vi "WhiteScreenTest_Startup.vi"() -> (0 "ErrorOut":errorcluster)   [LabVIEW 2018] (continued)
        n220 = Enqueue Element(queue=w531, element=cluster{"QElmnt":T47, "Data":variant} {"QElmnt"=enum."Spvsr_RfrshPnl", "Data"=variant} ("Cluster"), error in (no error)=w530) -> (error out=w529:errorcluster)  [unwired: 3 out]
        n221 = Variant To Data(error in=w529, type=w529, Variant=w532) -> (data=w533:errorcluster, error out=w525:errorcluster)
        n222 = Unbundle By Name(w533) -> ("code"=w526:i32)
        n223 = call "CheckForExistingErrorDialog.vi"("ErrorIn"=w525, "ErrorCodeIn"=w526) -> ("ErrorOut"=w523:errorcluster, "NoWndwFnd"=w522:bool, "ErrorCodeOut"=w524:i32)  [unwired: 7 in]
        n224 = call "PushToErrorHandler.vi"("ErrorIn"=w523, "ErrorLocation"="Error Handler") -> ("ErrorOut"=w538:errorcluster)  [unwired: 5 in]
        n225 = case shown="True" w522 {
          tunnel: w538 -> [w539 w547]
          tunnel: [w539 w546] -> w537
          tunnel: w536 -> [_ w545]
          tunnel: w535 -> [w540 w544]
          tunnel: [w540 w543] -> w534
          tunnel: w533 -> [_ w542]
          tunnel: w524 -> [_ w541]
          frame False {
          }
          frame True {
            n226 = case shown="-8998" w541 {
              tunnel: [w555 w564 w566 w573 w577 w584 w593] -> w546
              tunnel: w544 -> [w551 w560 w567 w572 w579 w589 w591]
              tunnel: [w550 w559 w568 w572 w580 w583 w591] -> w543
              tunnel: w547 -> [w556 w565 w566 w571 w577 w585 w594]
              tunnel: w542 -> [w554 w563 _ w574 _ w586 w595]
              tunnel: w545 -> [_ _ _ _ _ _ _]
              frame Default {
                # "-1 dictates that the message box does NOT time out"
                # "Default Error Case handles all error codes undefined by this structure."
                n227 = Bundle By Name(cluster=w551, "Stat.SysState"=SystemStateEnum."System Fault") -> (w550:T32)
                n228 = Unbundle By Name(w550) -> ("SMS"=w549:T36)
                n229 = call "LaunchSystemMessageDialogBox.vi"("ErrorToProcess"=w554, "SMS"=w549, "ErrorIn"=w556, "CorrAct"="Undocumented System Error, please record this information and contact the vendor.", "Timeout(ms)"=-1 ("Timeout (-1)")) -> ("ErrorOut"=w555:errorcluster)  [unwired: 6 in]
              }
              frame -8998 {
                # "-1 dictates that the message box does NOT time out"
                # "Default Error Case handles all error codes undefined by this structure."
                n230 = Bundle By Name(cluster=w560, "Stat.SysState"=SystemStateEnum."System Fault") -> (w559:T32)
                n231 = Unbundle By Name(w559) -> ("SMS"=w558:T36)
                n232 = call "LaunchSystemMessageDialogBox.vi"("ErrorToProcess"=w563, "SMS"=w558, "ErrorIn"=w565, "CorrAct"="The FPGAs are configured for an external 10 MHz reference clock. It doesn't look like that clock is working right.", "Timeout(ms)"=-1 ("Timeout (-1)")) -> ("ErrorOut"=w564:errorcluster)  [unwired: 6 in]
              }
              frame 5000 {
                # "Example User Defined Error Code.  Disable the Hardware and no Dialog Box"
                n233 = Bundle By Name(cluster=w567, "Stat.SysState"=SystemStateEnum."System Fault") -> (w568:T32)
              }
              frame 5998 {
                n234 = Unbundle By Name(w572) -> ("SMS"=w575:T36)
                n235 = call "LaunchSystemMessageDialogBox.vi"("ErrorToProcess"=w574, "SMS"=w575, "ErrorIn"=w571, "CorrAct"="Error Log Failure\n\n- There was an error writing to the Error Log File, please verify that the current user has read/write permissions to the <Users>\\My Documents & the <Users>\\Desktop folders" ("CorrAction"), "Timeout(ms)"=-1) -> ("ErrorOut"=w573:errorcluster)  [unwired: 6 in]
              }
              frame 5999 {
                n236 = Bundle By Name(cluster=w579, "Stat.SysState"=SystemStateEnum."System Error") -> (w580:T32)
              }
              frame 5100..5149 {
                # "Disable Hardware?"
                # "These error codes are reserved for Config File Reads"
                n237 = Bundle By Name(cluster=w589, "Stat.SysState"=SystemStateEnum."System Fault") -> (w583:T32)
                n238 = Unbundle By Name(w583) -> ("SMS"=w582:T36)
                n239 = call "LaunchSystemMessageDialogBox.vi"("ErrorToProcess"=w586, "SMS"=w582, "ErrorIn"=w585, "CorrAct"="Configuration File Read Error\n\n- One or more Configuration File Fields were not found or improperly loaded.\n- All System Hardware has been disabled\n- Launch the Configuration Panels and verify that all values have been correctly entered\n- Reinitialize the Hardware" ("CorrAction"), "Timeout(ms)"=-1 ("Timeout")) -> ("ErrorOut"=w584:errorcluster)  [unwired: 6 in]
              }
              frame 5150..5199 {
                # "No need to disable hardware here"
                # "These error codes are reserved for Config File Writes"
                n240 = Unbundle By Name(w591) -> ("SMS"=w592:T36)
                n241 = call "LaunchSystemMessageDialogBox.vi"("ErrorToProcess"=w595, "SMS"=w592, "ErrorIn"=w594, "CorrAct"="Configuration File Write Error\n\n- One or more Configuration File Fields were not found or specified incorrectly.\n- Launch the Configuration Panels and verify that all values have been correctly entered" ("CorrAction"), "Timeout(ms)"=-1 ("Timeout")) -> ("ErrorOut"=w593:errorcluster)  [unwired: 6 in]
              }
            }
          }
        }
      }
      frame "Spvsr_Config" {
        # "Opens the Configuration Panel"
        n242 = Current VI's Path() -> (path=w602:path)
        n243 = call "SetVIWindowTransparency.vi"("VIPath"=w602, "ErrorIn"=w603) -> ("ErrorOut"=w601:errorcluster)  [unwired: 9 in]
        n244 = call "ConfigPanel.vi"("ErrorIn"=w601, "ClusterIn"=w604) -> ("ErrorOut"=w597:errorcluster, "ClusterOut"=w598:T32)  [unwired: 8 out]
        n245 = Current VI's Path() -> (path=w599:path)
        n246 = call "RestoreVIWindowTransparency.vi"("VIPath"=w599, "ErrorIn"=w597) -> ("ErrorOut"=w600:errorcluster)  [unwired: 9 in]
      }
      frame "Spvsr_FPConfig" {
        w647 = ScaleMeasure."50" ("ScaleMeasure")
        w644 = ext 1.0 ("Scale_In_RT")
        w645 = fxp<+/-,30,30> 536870911.0 ("Scale_NoiseFloor")
        # "Don't start other loops if paths are bad."
        n247 = disable-structure shown="Enabled" {
          disable-tunnel: w609 -> [w668 _]
          disable-tunnel: [w667 T41 {"#NoiseSums"=1, "Max_df"=1, "AvgAvg"=FALSE, "#Avg"=1, "AutoCenter"=FALSE, "Inclin"={"Vmin"=0.0, "Vmax"=0.0, "Angle_min"=0.0, "Angle_max"=0.0, "Offset"=0.0, "Pos_Neg"=FALSE}, "1"={"Cal_"={"Fine"=0.000213623046875, "Coarse_"=4194303.0}, "Beac"={"Fine"=4194303.0, "Coarse_"=1.0}, "Scale"={"Step4"=10000.0, "Step5"=4194303.0, "Step6"=1.0, "Step7"=10000.0}, "Offset"=0.0, "Scale_Noise"=4194303.0, "Scale_Step1"=65535.0, "Scale_In_RT"=1.0, "ScaleMeas"=0.999969482421875, "FreqsToRemove"=[0, 1633], "Width"=[0, 1633], "ScaleMeasEnum"=enum."50", "FilterEnab"=enum."Step 1"}, "2"={"Cal_"={"Fine"=0.000213623046875, "Coarse_"=4194303.0}, "Beac"={"Fine"=0.000213623046875, "Coarse_"=4194303.0}, "Scale"={"Step4"=0.0, "Step5"=4194303.0, "Step6"=1.0, "Step7"=10000.0}, "Offset"=0.0, "Scale_Noise"=4194303.0, "Scale_Step1"=65535.0, "Scale_In_RT"=1.0, "ScaleMeas"=0.999969482421875, "FreqsToRemove"=[0, 1633], "Width"=[0, 1633], "ScaleMeasEnum"=enum."50", "FilterEnab"=enum."Step 1"}, "3"={"Cal_"={"Fine"=0.000213623046875, "Coarse_"=4194303.0}, "Beac"={"Fine"=0.000213623046875, "Coarse_"=4194303.0}, "Scale"={"Step4"=0.0, "Step5"=4194303.0, "Step6"=1.0, "Step7"=10000.0}, "Offset"=0.0, "Scale_Noise"=4194303.0, "Scale_Step1"=65535.0, "Scale_In_RT"=1.0, "ScaleMeas"=0.999969482421875, "FreqsToRemove"=[0, 1633], "Width"=[0, 1633], "ScaleMeasEnum"=enum."50", "FilterEnab"=enum."Step 1"}, "4"={"Cal_"={"Fine"=0.000213623046875, "Coarse_"=4194303.0}, "Beac"={"Fine"=0.000213623046875, "Coarse_"=4194303.0}, "Scale"={"Step4"=0.0, "Step5"=4194303.0, "Step6"=1.0, "Step7"=10000.0}, "Offset"=0.0, "Scale_Noise"=4194303.0, "Scale_Step1"=1.0, "Scale_In_RT"=10000.0, "ScaleMeas"=0.999969482421875, "FreqsToRemove"=[0, 1633], "Width"=[0, 1633], "ScaleMeasEnum"=enum."50", "FilterEnab"=enum."Step 1"}, "Target to Probe"=enum."4", "SNR_Thresh"=1.0, "Paths"={"CfgFile"=path "", "LogFolder"=path "", "LogFile"=path "", "NAS path"=path "", "ThreshFile"=path "", "RedunFolder"=path ""}, "Connex_Location"="", "SimulateFPGA"=FALSE} ("FP_User")] -> w608
          frame Enabled {
            # "12/14/2020"
            n248 = Unbundle By Name(w668) -> ("Config.FP_User"=w667:T41)
          }
          frame Disabled {
          }
        }
        n249 = Unbundle By Name("Scale") -> ("Measure"=w631:fxp<+/-,16,1>, "Step1"=w632:fxp<+/-,17,17>, "Scale"=w633:T5)
        n250 = call "RootExists.vi"("path"="NAS path") -> ("file or folder exists?"=w611:bool)  [unwired: 10 in]
        n251 = Negate(x="Shift Cal") -> (-x=w626:T11)
        n252 = Negate(x="Shift Beac") -> (-x=w625:T11)
        n253 = Not(x=w611) -> (.not. x?=→"Logging to NAS":bool)
        n254 = Bundle By Name(cluster=w608, "1.ScaleMeas"=w631, "1.Scale_Step1"=w632, "1.Scale"=w633, "1.ScaleMeasEnum"=w647, "AvgAvg"="AvgAvg", "1.FreqsToRemove"="FreqsToRemove", "1.Width"="Width [bins]", "1.Cal_"=w626, "1.Beac"=w625, "1.FilterEnab"="FilterEnable", "1.Scale_Noise"=w645, "1.Scale_In_RT"=w644, "#NoiseSums"=u32 86400 ("#NoiseSums to log"), "AutoCenter"="AutoCenter", "Target to Probe"="Target to Probe", "#Avg"=u16 150 ("#Avg in FPGA"), "SNR_Thresh"="SNR_Thresh", "Inclin"="Inclin", "Paths.RedunFolder"="base path", "Paths.LogFolder"="base path", "Paths.NAS path"="NAS path", "Paths.ThreshFile"="ThreshFile", "Connex_Location"="Location", "Max_df"="MaxTrackRate", "SimulateFPGA"="SimulateFPGA") -> (w656:T41)
        n255 = Build Array("base path", "ThreshFile") -> (w629:path[])
        n256 = Select(t=enum32{"Auto", "Manual"}."Auto" ("FreqShiftTab"), s="AutoCenter", f=enum32{"Auto", "Manual"}."Manual" ("FreqShiftTab")) -> (s? t:f=→"FreqShiftTab_72Co" →"FreqShiftTab_84Co":enum32{"Auto", "Manual"})
        n257 = for {
          tunnel: w629 -> [w679] mode=indexing
          tunnel: [w677] -> w628 mode=indexing
          n258 = call "RootDoesntExist.vi"("base path in"=w679) -> ("String"=w678:string)  [unwired: 10 in]
          n259 = call "RootExists.vi"("path"=w679) -> ("file or folder exists?"=w677:bool)  [unwired: 10 in]
          n260 = case shown="False" w677 {
            tunnel: w678 -> [w680 _]
            frame False {
              n261 = One Button Dialog(message=w680) -> ()  [unwired: 1 in, 1 out]
            }
            frame True {
            }
          }
        }
        n262 = Unbundle By Name(w656) -> ("2"=w655:T42)
        n263 = Bundle By Name(cluster=w655, "ScaleMeas"=w631, "Scale_Step1"=w632, "Scale"=w633, "ScaleMeasEnum"=w647, "FreqsToRemove"="FreqsToRemove", "Width"="Width [bins]", "FilterEnab"="FilterEnable", "Scale_Noise"=w645, "Scale_In_RT"=w644, "Cal_"=w626, "Beac"=w625) -> (w657:T42)
        n264 = Bundle By Name(cluster=w656, "2"=w657) -> (w650:T41)
        n265 = Negate(x="Shift Cal 3") -> (-x=w624:T11)
        n266 = Negate(x="Shift Beac 3") -> (-x=w623:T11)
        n267 = Unbundle By Name(w650) -> ("3"=w654:T42)
        n268 = Bundle By Name(cluster=w654, "ScaleMeas"=w631, "Scale_Step1"=w632, "Scale"=w633, "ScaleMeasEnum"=w647, "FreqsToRemove"="FreqsToRemove 2", "Width"="Width 2 [bins]", "FilterEnab"="FilterEnable", "Scale_Noise"=w645, "Scale_In_RT"=w644, "Cal_"=w624, "Beac"=w623) -> (w653:T42)
        n269 = And Array Elements(Boolean array=w628) -> (logical AND=w627:bool)
        n270 = Bundle By Name(cluster=w650, "3"=w653) -> (w649:T41)
        n271 = Unbundle By Name(w649) -> ("4"=w651:T42)
        n272 = Bundle By Name(cluster=w651, "ScaleMeas"=w631, "Scale_Step1"=w632, "Scale"=w633, "ScaleMeasEnum"=w647, "FreqsToRemove"="FreqsToRemove 2", "Width"="Width 2 [bins]", "FilterEnab"="FilterEnable", "Scale_Noise"=w645, "Scale_In_RT"=w644, "Cal_"=w624, "Beac"=w623) -> (w652:T42)
        n273 = Bundle By Name(cluster=w649, "4"=w652) -> (w648:T41)
        n274 = Bundle By Name(cluster=w609, "Config.FP_User"=w648) -> (w619:T32)
        n275 = Bundle By Name(cluster=w619, "Config.FP_User.Max_df"=u32 1) -> (w618:T32)
        n276 = case shown="True" w627 {
          tunnel: w666 -> [w670 w676]
          tunnel: w619 -> [_ w671]
          tunnel: w664 -> [_ w675]
          tunnel: [w670 w674] -> w660
          tunnel: w659 -> [_ w673]
          tunnel: w635 -> [_ w672]
          frame False {
          }
          frame True {
            n277 = call "Send_Front_Panel_Config_to_Loops.vi"("ClusterIn"=w671, "Log_Q"=w672, "error in (no error)"=w676, "Noise_Q"=w673, "Tones_Q"=w675) -> ("error out"=w674:errorcluster)  [unwired: 6 in]
          }
        }
        n278 = call "WriteConfigFile.vi"("ErrorIn"=w660, "ClusterIn"=w618) -> ("ErrorOut"=w665:errorcluster)  [unwired: 1 in, 8 out]
        "Auto Center" <- "AutoCenter"
      }
      frame "Spvsr_AlarmCfg" {
        # "We send alarm configurations to AI and TC. The voltage and\ntemp indicators are color-coded red & yellow if there are \nalarms or wanings. These are calculated in the AI loops."
        # "We need to send the alarm configuration to the log loop because that is\nwhere we will check the alarm statuses. It's the only place where we can find\nthe data from AI, TC, TE, ADAM, and spectra."
        n279 = Unbundle By Name(w693) -> ("Config.FP_User.Paths.ThreshFile"=w692:path)
        n280 = Bundle By Name(cluster=w693, "Alarm"="AlarmSettings") -> (w696:T32)
        n281 = Flatten To XML(anything="AlarmSettings") -> (xml string=w695:string)
        n282 = call-poly <vilib>:"Write to XML File.vi"("error in (no error)"=w694, "XML Input"=w695, "XML File Path"=w692) -> ("error out"=w691:errorcluster)  [unwired: 6 in, 2 out]
        n283 = To Variant(anything="AlarmSettings") -> (Variant=w682:variant)
        n284 = To Variant(anything="AlarmSettings") -> (Variant=w686:variant)
        n285 = Bundle By Name(cluster=cluster{"Enum":T30, "Data":variant} {"Enum"=enum."Log_CfgAlarm", "Data"=variant} ("element"), "Data"=w686) -> (w687:cluster{"Enum":T30, "Data":variant})
        n286 = Bundle By Name(cluster=cluster{"Enum":T53, "Var":variant} {"Enum"=enum."AI_Alarm", "Var"=variant}, "Var"=w682) -> (w683:cluster{"Enum":T53, "Var":variant})
        n287 = Enqueue Element(queue=w689, element=w687, error in (no error)=w691) -> (error out=w690:errorcluster)  [unwired: 1 in, 2 out]
        n288 = for {
          tunnel: string[] ["AI", "TC"] ("name (unnamed)") -> [w704] mode=indexing
          tunnel: w683 -> [w697]
          n289 = Obtain Queue(max queue size (-1, unlimited)=100, name (unnamed)=w704, element data type=w697) -> (queue out=w702:refnum<queue>, error out=w703:errorcluster)  [unwired: 2 in, 1 out]
          n290 = Enqueue Element(queue=w702, element=w697, error in (no error)=w703) -> (queue out=w700:refnum<queue>, error out=w701:errorcluster)  [unwired: 1 in, 1 out]
          n291 = Release Queue(queue=w700, error in (no error)=w701) -> (error out=w699:errorcluster)  [unwired: 1 in, 2 out]
          n292 = call "PushToErrorHandler.vi"("ErrorIn"=w699, "ErrorLocation"="SendAlarmToAI_orTC") -> ()  [unwired: 5 in, 1 out]
        }
      }
      frame "Spvsr_DigitzOffs" {
        w714 = fxp<+/-,16,16> 0.0 ("fixed-point type")
        n293 = local read "84 GHz"() -> (w722:T3)
        n294 = local read "72 GHz"() -> (w723:T3)
        n295 = Unbundle By Name(w723) -> ("MeasMean0"=w719:dbl, "MeasMean1"=w717:dbl)
        n296 = Unbundle By Name(w722) -> ("MeasMean0"=w716:dbl, "MeasMean1"=w715:dbl)
        n297 = Negate(x=w719) -> (-x=w709:dbl)
        n298 = Negate(x=w717) -> (-x=w708:dbl)
        n299 = Negate(x=w716) -> (-x=w707:dbl)
        n300 = Negate(x=w715) -> (-x=w706:dbl)
        n301 = To Fixed-Point(fixed-point type=w714, number=w709) -> (fixed-point=w718:fxp<+/-,16,16>)
        "Digitizer Offset 72 Co" <- w718
        n302 = To Fixed-Point(fixed-point type=w714, number=w708) -> (fixed-point=w712:fxp<+/-,16,16>)
        "Digitizer Offset 72 X" <- w712
        n303 = To Fixed-Point(fixed-point type=w714, number=w707) -> (fixed-point=w711:fxp<+/-,16,16>)
        "Digitizer Offset 84 Co" <- w711
        n304 = To Fixed-Point(fixed-point type=w714, number=w706) -> (fixed-point=w710:fxp<+/-,16,16>)
        "Digitizer Offset 84 x" <- w710
        n305 = Bundle By Name(cluster=w720, "Config.FP_User.1.Offset"=w718, "Config.FP_User.2.Offset"=w712, "Config.FP_User.3.Offset"=w711, "Config.FP_User.4.Offset"=w710) -> (w721:T32)
      }
      frame "FP_AO_ctrl" {
        w746 = 5.0
        w747 = 0.0
        w741 = cluster{"Enum":T55, "Data":variant} {"Enum"=enum."AO_Write", "Data"=variant}
        # "As defined in Wiring_Pinout Diagrams_DRAFT_20171207.xlsx\nfrom Nick Tarasenko.\nLuke 12-12-2017"
        # "Cal tones: 5 is on, 0 is off"
        # "Noise: 0 is on, 5 is off"
        n306 = Select(t=w747, s="noise_ctrl", f=w746) -> (s? t:f=w745:dbl)
        n307 = Select(t=w746, s="72GHz_ctrl", f=w747) -> (s? t:f=w744:dbl)
        n308 = Select(t=w746, s="84GHz_ctrl", f=w747) -> (s? t:f=w743:dbl)
        n309 = Obtain Queue(max queue size (-1, unlimited)=100, name (unnamed)="AO", element data type=w741, error in (no error)=w748) -> (queue out=w751:refnum<queue>, error out=w737:errorcluster)  [unwired: 1 in, 1 out]
        n310 = Build Array("noise_ctrl", "72GHz_ctrl", "84GHz_ctrl") -> (w726:bool[])
        n311 = Build Array(w745, w744, w743) -> (w742:dbl[])
        n312 = To Variant(anything=w742) -> (Variant=w730:variant)
        n313 = Bundle By Name(cluster=w741, "Data"=w730) -> (w740:cluster{"Enum":T55, "Data":variant})
        n314 = Enqueue Element(queue=w751, element=w740, error in (no error)=w737) -> (queue out=w736:refnum<queue>, error out=w738:errorcluster)  [unwired: 1 in, 1 out]
        n315 = To Variant(anything=w726) -> (Variant=w725:variant)
        n316 = Release Queue(queue=w736, error in (no error)=w738) -> (error out=w735:errorcluster)  [unwired: 1 in, 2 out]
        n317 = Bundle By Name(cluster=cluster{"Enum":T30, "Data":variant} {"Enum"=enum."Log_DO", "Data"=variant} ("element"), "Data"=w725) -> (w731:cluster{"Enum":T30, "Data":variant})
        n318 = Enqueue Element(queue=w733, element=w731, timeout in ms (-1)=10, error in (no error)=w735) -> (error out=w734:errorcluster)  [unwired: 2 out]
      }
      frame "Spvsr_ScaleGraphs" {
        w786 = 1000000.0 ("y")
        w783 = 10.0 ("y")
        # "This was a local variable tied to Frequency Shift Enable, before the control was changed to a constant. Luke 6-1-2018"
        n319 = local read "BeaconShift 3"() -> (w765:dbl)
        n320 = local read "BeaconShift 2"() -> (w799:dbl)
        n321 = local read "BeaconShift 4"() -> (w763:dbl)
        n322 = local read "BeaconShift"() -> (w795:dbl)
        n323 = local read "Peak Location Beacon"() -> (w781:dbl)
        n324 = local read "Peak Location Cal"() -> (w782:dbl)
        n325 = local read "Peak Location Beacon 2"() -> (w801:dbl)
        n326 = local read "Peak Location Cal 2"() -> (w802:dbl)
        n327 = local read "Peak Location Beacon 3"() -> (w761:dbl)
        n328 = local read "Peak Location Cal 3"() -> (w760:dbl)
        n329 = local read "Peak Location Beacon 4"() -> (w759:dbl)
        n330 = local read "Peak Location Cal 4"() -> (w758:dbl)
        n331 = local read "CalShift 3"() -> (w764:dbl)
        n332 = local read "CalShift 2"() -> (w800:dbl)
        n333 = local read "CalShift"() -> (w796:dbl)
        n334 = local read "CalShift 4"() -> (w762:dbl)
        n335 = control-ref of="NoiseFloor"() -> (w756:refnum<vi>)
        n336 = control-ref of="NoiseFloor 2"() -> (w754:refnum<vi>)
        n337 = control-ref of="NoiseFloor 3"() -> (w753:refnum<vi>)
        n338 = control-ref of="NoiseFloor 4"() -> (w752:refnum<vi>)
        n339 = local read "df (Hz)"() -> (w777:dbl)
        n340 = Build Array(w795, w796, w799, w800, w765, w764, w763, w762) -> (w790:dbl[])
        n341 = Build Array(w756, w754, w753, w752) -> (w755:refnum<vi>[])
        n342 = for {
          tunnel: [w833] -> w772
          tunnel: w790 -> [w835] mode=indexing
          tunnel: TRUE -> [w829]
          tunnel: [w828] -> w771 mode=indexing
          n343 = local read "df (Hz)"() -> (w836:dbl)
          n344 = Divide(x=w836, y=1000000.0) -> (x/y=w833:dbl)
          n345 = Divide(x=w835, y=1000000.0) -> (x/y=w831:dbl)
          n346 = Select(t=w831, s=w829, f=0.0) -> (s? t:f=w828:dbl)
        }
        n347 = Build Array(w781, w782, w801, w802, w761, w760, w759, w758) -> (w791:dbl[])
        n348 = for {
          tunnel: w777 -> [w805]
          tunnel: u8 0 ("Noise Floor") -> [w804]
          tunnel: w755 -> [w803] mode=indexing
          n349 = property class="WFGraph (strict)"(reference=w803, "YScale.Mapping Mode"=w804, "XScale.Multiplier"=w805) -> ()  [unwired: 1 in, 2 out]
        }
        n350 = case shown="True" "AutoScale Y Noise" {
          tunnel: w755 -> [_ w806]
          frame False {
          }
          frame True {
            n351 = for {
              tunnel: w806 -> [w808] mode=indexing
              n352 = property class="WFGraph (strict)"(reference=w808, "YScale.ScaleFit"=u8 1 ("Y Scale.Scale Fit")) -> ()  [unwired: 1 in, 2 out]
            }
          }
        }
        n353 = Add(x=w791, y=w783) -> (x+y=w784:dbl[])
        n354 = Subtract(x=w791, y=w783) -> (x-y=w785:dbl[])
        n355 = Divide(x=w784, y=w786) -> (x/y=w788:dbl[])
        n356 = Divide(x=w785, y=w786) -> (x/y=w789:dbl[])
        n357 = control-ref of="All Spectrums"() -> (w773:refnum<vi>)
        n358 = Index Array(array=w771) -> (element=w770:dbl)  [unwired: 1 in]
        n359 = control-ref of="Beacon 2"() -> (w797:refnum<vi>)
        n360 = control-ref of="Cal 2"() -> (w798:refnum<vi>)
        n361 = control-ref of="Beacon 3"() -> (w769:refnum<vi>)
        n362 = control-ref of="Beacon"() -> (w780:refnum<vi>)
        n363 = control-ref of="Cal"() -> (w778:refnum<vi>)
        n364 = control-ref of="Cal 3"() -> (w768:refnum<vi>)
        n365 = control-ref of="Cal 4"() -> (w766:refnum<vi>)
        n366 = control-ref of="Beacon 4"() -> (w767:refnum<vi>)
        n367 = property class="WFGraph (strict)"(reference=w773, "XScale.Multiplier"=w772, "XScale.Offset"=w770) -> ()  [unwired: 1 in, 2 out]
        n368 = Build Array(w780, w778, w797, w798, w769, w768, w767, w766) -> (w792:refnum<vi>[])
        n369 = for {
          tunnel: w792 -> [w840] mode=indexing
          tunnel: u8 0 ("Tones") -> [w839]
          tunnel: w772 -> [w838]
          tunnel: w771 -> [w837] mode=indexing
          n370 = property class="WFGraph"(reference=w840, "YScale.Mapping Mode"=w839, "XScale.Multiplier"=w838, "XScale.Offset"=w837) -> ()  [unwired: 1 in, 2 out]
        }
        n371 = for {
          tunnel: w792 -> [w816] mode=indexing
          tunnel: "Zoom On Peak" -> [w815]
          tunnel: w788 -> [w814] mode=indexing
          tunnel: w789 -> [w813] mode=indexing
          tunnel: [w812] -> _
          n372 = case shown="True" w815 {
            tunnel: w816 -> [w821 w823]
            tunnel: w814 -> [w819 _]
            tunnel: w813 -> [w818 _]
            tunnel: [w817 w822] -> w812
            frame True {
              n373 = property class="WFGraph"(reference=w821, "XScale.ScaleFit"=u8 0 ("X Scale.Scale Fit"), "XScale.Maximum"=w819, "XScale.Minimum"=w818) -> (error out=w817:errorcluster)  [unwired: 1 in, 1 out]
            }
            frame False {
              n374 = disable-structure shown="Disabled" {
                disable-tunnel: w823 -> [w826 _]
                disable-tunnel: [w824 errorcluster {"status"=FALSE, "code"=0, "source"=""} ("error out")] -> w822
                frame Enabled {
                  n375 = property class="WFGraph"(reference=w826, "XScale.ScaleFit"=u8 2 ("X Scale.Scale Fit")) -> (error out=w824:errorcluster)  [unwired: 1 in, 1 out]
                }
                frame Disabled {
                }
              }
            }
          }
        }
        n376 = case shown="True" "AutoScale Y Tones" {
          tunnel: w792 -> [_ w809]
          frame False {
          }
          frame True {
            n377 = for {
              tunnel: w809 -> [w810] mode=indexing
              n378 = property class="WFGraph"(reference=w810, "YScale.ScaleFit"=u8 1 ("Y Scale.Scale Fit")) -> ()  [unwired: 1 in, 2 out]
            }
          }
        }
      }
      frame "Spvsr_TrackRate" {
        n379 = Bundle By Name(cluster=w842, "Stat.TrackRate"=FALSE) -> (w843:T32)
      }
      frame "Spvsr_AutoCenter" {
        w845 = FALSE  # Stat.AutoCentr
        n380 = Bundle By Name(cluster=w846, "Stat.AutoCentr"=w845) -> (w847:T32)
      }
      frame "Spvsr_RestartWarn" {
        n381 = One Button Dialog(message="When changing file paths, the change will not be implemented until the program is restarted.\n\nWhen changing the \"Connex Location\", the change will not be written to the data log header until a new file is made (either at midnight, or upon restarting.)") -> ()  [unwired: 1 in, 1 out]
      }
      frame "Spvsr_ChkTime" {
        # "Reset peak tracker to default 10 minutes after user changes it."
        n382 = Unbundle By Name(w866) -> ("Stat.AutoCentr"=w858:bool, "Stat.TrackRate"=w868:bool)
        n383 = call "Elapsed Time4"("Time Target (s)"=600.0, "Reset"=w868, "error in (no error)"=w869) -> ("Elapsed Time (s)"=w864:dbl, "Time has Elapsed"=w867:bool, "error out"=w865:errorcluster)  [unwired: 9 in, 5 out]
        n384 = case shown="True" w867 {
          tunnel: w866 -> [w887 w895]
          tunnel: [w887 w894] -> w855
          tunnel: w865 -> [w888 w892]
          tunnel: [w888 w889] -> w857
          tunnel: w864 -> [_ _]
          frame False {
          }
          frame True {
            n385 = control-ref of="MaxTrackRate"() -> (w891:refnum<vi>)
            n386 = property class="DigNum (strict)"(reference=w891, error in=w892, "Val(Sgnl)"=u32 1 ("Value (Signaling)")) -> (error out=w889:errorcluster)  [unwired: 1 out]
            n387 = Bundle By Name(cluster=w895, "Stat.TrackRate"=TRUE) -> (w894:T32)
          }
        }
        n388 = call "Elapsed Time5"("Time Target (s)"=600.0, "Reset"=w858, "error in (no error)"=w857) -> ("Elapsed Time (s)"=w861:dbl, "Time has Elapsed"=w859:bool, "error out"=w860:errorcluster)  [unwired: 9 in, 5 out]
        n389 = case shown="True" w859 {
          tunnel: w855 -> [w878 w886]
          tunnel: [w878 w885] -> w854
          tunnel: w860 -> [w879 w883]
          tunnel: [w879 w881] -> w856
          tunnel: w861 -> [_ _]
          frame False {
          }
          frame True {
            n390 = control-ref of="AutoCenter"() -> (w882:refnum<vi>)
            n391 = property class="Bool (strict)"(reference=w882, error in=w883, "Val(Sgnl)"=TRUE ("Value (Signaling)")) -> (error out=w881:errorcluster)  [unwired: 1 out]
            n392 = Bundle By Name(cluster=w886, "Stat.AutoCentr"=TRUE ("Stat.TrackRate")) -> (w885:T32)
          }
        }
        n393 = call "Elapsed Time3"("Time Target (s)"=2.0, "error in (no error)"=w856) -> ("Time has Elapsed"=w875:bool, "error out"=w852:errorcluster)  [unwired: 10 in, 6 out]
        n394 = Select(t=cluster{"QElmnt":T47, "Data":variant}[] [{"QElmnt"=enum."Spvsr_ScaleGraphs", "Data"=variant}, {"QElmnt"=enum."Spvsr_ChkTime", "Data"=variant}], s=w875, f=cluster{"QElmnt":T47, "Data":variant}[] [{"QElmnt"=enum."Spvsr_ChkTime", "Data"=variant}]) -> (s? t:f=w877:cluster{"QElmnt":T47, "Data":variant}[])
        n395 = for {
          tunnel: w877 -> [w898] mode=indexing
          tunnel: w876 -> [w897]
          shift-right: [w896] -> w872
          shift-left: _ -> [_]
          n396 = Enqueue Element(queue=w897, element=w898) -> (error out=w896:errorcluster)  [unwired: 2 in, 2 out]
        }
        n397 = Wait Until Next ms Multiple(millisecond multiple=u32 100 ("milliseconds to wait")) -> ()  [unwired: 1 out]
        n398 = Merge Errors(w872, w852) -> (w853:errorcluster)
      }
      frame "Spvsr_About" {
        # "Pops up the About dialog box where you can enter version, customer, contact and any other information regarding the application."
        n399 = call "About.vi"("error in"=w902, "Timeout (ms)"=5000) -> ("error out"=w901:errorcluster)  [unwired: 9 out]
      }
      frame "Spvsr_Exit" {
        # "With the Exit Button, we exit this loop and push the HW Loops to close."
        n400 = call "Exit_All_Loops.vi"("error in (no error)"=w904, "10Hz_Q"=w903, "Noise_Q"=w906, "Tones_Q"=w907) -> ("error out"=w905:errorcluster)  [unwired: 7 in]
      }
    }
    "SPVSR_Count" <- w292
  }
  n401 = while {
    tunnel: w70 -> [w911]
    tunnel: w98 -> [w922]
    tunnel: [w916] -> w133
    shift-right: [w915] -> _
    shift-left: T24 {"Alarms"={"Green"=FALSE, "Rx_Yell"=FALSE, "Cx_Yell"=FALSE, "Red"=FALSE, "Source"=""}, "Spectrum 1"=[], "Spectrum 2"=[], "Spectrum 3"=[], "Spectrum 4"=[], "HistoryWeighting"=0.0, "NoiseFloorSums"={"1"=0.0, "2"=0.0, "3"=0.0, "4"=0.0}, "PwrHist"={"72Co"={"Cal"=0.0, "Cal Smooth"=0.0, "Beac"=0.0, "Beac Smooth"=0.0, "NoiseFloorSum"=0.0, "NoiseFloorSum Smooth"=0.0}, "72X"={"Cal"=0.0, "Cal Smooth"=0.0, "Beac"=0.0, "Beac Smooth"=0.0, "NoiseFloorSum"=0.0, "NoiseFloorSum Smooth"=0.0}, "84Co"={"Cal"=0.0, "Cal Smooth"=0.0, "Beac"=0.0, "Beac Smooth"=0.0, "NoiseFloorSum"=0.0, "NoiseFloorSum Smooth"=0.0}, "84X"={"Cal"=0.0, "Cal Smooth"=0.0, "Beac"=0.0, "Beac Smooth"=0.0, "NoiseFloorSum"=0.0, "NoiseFloorSum Smooth"=0.0}}} -> [w914]
    tunnel: w92 -> [w913]
    i -> [w912]
    stop <- w917 stop-if-true
    # "Front panel updates"
    n402 = call "PushToErrorHandler.vi"("ErrorIn"=w922, "ErrorLocation"="FP") -> ("ErrorOut"=w924:errorcluster)  [unwired: 5 in]
    n403 = Get Queue Status(queue=w911) -> (# elements in queue=→"# in FP queue":i32)  [unwired: 2 in, 7 out]
    n404 = Dequeue Element(queue=w911, error in (no error)=w924) -> (queue out=w918:refnum<queue>, element=w923:cluster{"Enum":T28, "Data":variant}, error out=w919:errorcluster)  [unwired: 1 in, 1 out]
    n405 = Unbundle(w923) -> ("Enum"=w921:T28, "Data"=w920:variant)
    n406 = case shown="\"FP_Tone\"" w921 {
      tunnel: w920 -> [_ _ w955 w1132 w1179 w1189 w1227 w1263 _ w1350 _]
      tunnel: w919 -> [w936 w938 w948 w1133 w1181 w1191 w1229 w1264 w1284 w1351 w1364]
      tunnel: w918 -> [_ _ w946 _ _ _ _ _ _ _ w1365]
      tunnel: [_ _ _ _ _ _ _ _ _ _ TRUE] -> w917
      tunnel: [w936 w938 w948 w1133 w1182 w1190 w1228 w1237 w1284 w1338 w1363] -> w916
      tunnel: [w937 w939 w949 w1126 w1168 w1183 w1202 w1255 w1283 w1352 w1362] -> w915
      tunnel: w914 -> [w937 w939 w950 w1127 w1168 w1183 w1202 w1255 w1283 w1352 w1362]
      tunnel: w913 -> [_ _ _ _ _ _ _ _ _ _ _]
      frame "FP_Init", Default {
        w926 = cluster{dbl, dbl, dbl}[] [] ("History Data")
        w927 = T72 [] ("History Data")
        n407 = control-ref of="Power History 72 Co"() -> (w935:refnum<vi>)
        n408 = control-ref of="Power History 72 X"() -> (w934:refnum<vi>)
        n409 = control-ref of="Power History 84 Co"() -> (w933:refnum<vi>)
        n410 = control-ref of="Power History 84 X"() -> (w932:refnum<vi>)
        n411 = control-ref of="Freq History 72 Co"() -> (w931:refnum<vi>)
        n412 = control-ref of="Freq History 72 X"() -> (w930:refnum<vi>)
        n413 = control-ref of="Freq History 84 Co"() -> (w929:refnum<vi>)
        n414 = control-ref of="Freq History 84 X"() -> (w928:refnum<vi>)
        n415 = property class="WFChart (strict)"(reference=w935, "History Data"=w927) -> ()  [unwired: 1 in, 2 out]
        n416 = property class="WFChart (strict)"(reference=w934, "History Data"=w927) -> ()  [unwired: 1 in, 2 out]
        n417 = property class="WFChart (strict)"(reference=w933, "History Data"=w927) -> ()  [unwired: 1 in, 2 out]
        n418 = property class="WFChart (strict)"(reference=w932, "History Data"=w927) -> ()  [unwired: 1 in, 2 out]
        n419 = property class="WFChart (strict)"(reference=w931, "History Data"=w926) -> ()  [unwired: 1 in, 2 out]
        n420 = property class="WFChart (strict)"(reference=w930, "History Data"=w926) -> ()  [unwired: 1 in, 2 out]
        n421 = property class="WFChart (strict)"(reference=w929, "History Data"=w926) -> ()  [unwired: 1 in, 2 out]
        n422 = property class="WFChart (strict)"(reference=w928, "History Data"=w926) -> ()  [unwired: 1 in, 2 out]
      }
      frame "FP_Scale" {
        n423 = Unbundle By Name(w939) -> ("Spectrum 1"=w943:dbl[], "Spectrum 2"=w942:dbl[], "Spectrum 3"=w941:dbl[], "Spectrum 4"=w940:dbl[])
        n424 = Build Array(w943, w942, w941, w940) -> (→"All Spectrums":dbl[][])
      }
      frame "FP_Tone" {
        # "From Data_Send"
        n425 = local read "SNR_Thresh"() -> (w945:dbl)
        n426 = local read "AutoCenter"() -> (w947:bool)
        n427 = Variant To Data(error in=w948, type=cluster{"Target":T21, "1":T56} {"Target"=enum."1", "1"={"Cal"={"Shift_"=0.0, "Peak_ToFPGA"=-24999462.633451957, "MaxValue"=0.0, "MaxIndex"=0, "Tone"={"PkLocTrak"=0.0, "PkLocDisp"=0.0, "df_"=0.0, "ZoomPwr"=[], "Phase"=0.0, "PhaseOld"=0.0, "AboveThresh?"=FALSE, "MaxI"=0.0, "MaxQ"=0.0, "median"=0.0, "ISpect"=[], "QSpect"=[], "DeltaPhase"=0.0}, "TimeDomainI"=[], "TimeDomainQ"=array[12500 elements], "PwrSpectrum"=[], "RunningAvgFreq"=0.0, "ISpectPos"=[], "ISpectNeg"=[], "QSpectPos"=[], "QSpectNeg"=[], "10Hz_PwrSpectr"=[], "SNR"=0.0, "AliasWarn"=FALSE, "10Hz_Peak"=[], "ISpect+-"=[], "QSpect+-"=[], "TimeStamp"=timestamp(0 s since 1904-01-01), "I_Index"=array[12500 elements], "Q_Index"=array[12500 elements], "10MHz"=FALSE}, "Beac"={"Shift_"=0.0, "Peak_ToFPGA"=-24999462.633451957, "MaxValue"=0.0, "MaxIndex"=0, "Tone"={"PkLocTrak"=0.0, "PkLocDisp"=0.0, "df_"=0.0, "ZoomPwr"=[], "Phase"=0.0, "PhaseOld"=0.0, "AboveThresh?"=FALSE, "MaxI"=0.0, "MaxQ"=0.0, "median"=0.0, "ISpect"=[], "QSpect"=[], "DeltaPhase"=0.0}, "TimeDomainI"=[], "TimeDomainQ"=array[12500 elements], "PwrSpectrum"=[], "RunningAvgFreq"=0.0, "ISpectPos"=[], "ISpectNeg"=[], "QSpectPos"=[], "QSpectNeg"=[], "10Hz_PwrSpectr"=[], "SNR"=0.0, "AliasWarn"=FALSE, "10Hz_Peak"=[], "ISpect+-"=[], "QSpect+-"=[], "TimeStamp"=timestamp(0 s since 1904-01-01), "I_Index"=array[12500 elements], "Q_Index"=array[12500 elements], "10MHz"=FALSE}, "Time"=[], "Saturat"={"MeasMean0"=0.0, "MeasMean1"=0.0, "MeasMax"=0.0, "1_Max"=0.0, "4_Max"=0.0, "5_Max"=0.0, "6_Max"=0.0, "7_Max"=0.0}}} ("cluster"), Variant=w955) -> (data=w953:cluster{"Target":T21, "1":T56})  [unwired: 1 out]
        n428 = Unbundle(w953) -> ("Target"=w952:T21, "1"=w951:T56)
        n429 = case shown="\"2\", Default" w952 {
          tunnel: w951 -> [w1012 w1042 w1091 w1122]
          tunnel: w950 -> [w1001 w1029 w1076 w1108]
          tunnel: [w1002 w1033 w1084 w1115] -> w949
          tunnel: w947 -> [w997 _ w1079 _]
          tunnel: w946 -> [_ _ _ w1094]
          tunnel: w945 -> [w978 _ w1067 _]
          frame "1" {
            # "Update all history charts"
            # "All freq locations displayed as positive."
            # "df is the same for cal & beac"
            n430 = Unbundle By Name(w1012) -> ("Cal"=w1011:T57, "Saturat"=→"72 GHz":T3, "Beac"=w1009:T57)
            n431 = Unbundle By Name(w1009) -> ("10Hz_PwrSpectr"=→"Beacon 10Hz":dbl[][], "Shift_"=w1008:dbl, "MaxValue"=w995:dbl, "Tone"=w972:T58, "TimeDomainI"=→"TimeDomainBeac":ext[], "PwrSpectrum"=w980:dbl[], "ISpectPos"=→"IPos":dbl[], "ISpectNeg"=→"INeg":dbl[], "QSpectPos"=→"QPos":dbl[], "QSpectNeg"=→"QNeg":dbl[], "Tone.ZoomPwr"=→"Power":dbl[], "SNR"=w983:dbl, "TimeDomainI"=→"72 Co Beac I":ext[], "TimeDomainQ"=→"72 Co Beac Q":ext[], "I_Index"=→"Co I_Index":ext[])
            "Channel Power Beac" <- w995
            "SNR" <- w983
            "Signal-to-Noise Ratio on 72 Co" <- w983
            n432 = Unbundle By Name(w1011) -> ("10Hz_PwrSpectr"=→"Cal 10Hz":dbl[][], "Shift_"=w1010:dbl, "MaxValue"=w968:dbl, "Tone"=w988:T58, "TimeDomainI"=→"TimeDomainCal":ext[], "PwrSpectrum"=→"Cal":dbl[])
            "Channel Power Cal" <- w968
            "MaxValue_Cal_72Co" <- w968
            n433 = Unbundle By Name(w972) -> ("PkLocDisp"=w1006:dbl)
            n434 = Negate(x=w1010) -> (-x=w969:dbl)
            "CalShift" <- w969
            n435 = Negate(x=w1008) -> (-x=w971:dbl)
            "BeaconShift" <- w971
            n436 = Unbundle By Name(w988) -> ("PkLocTrak"=w1007:dbl, "df_"=→"df (Hz)":dbl)
            n437 = Negate(x=w1006) -> (-x=w970:dbl)
            "Peak Location Beacon" <- w970
            n438 = Unbundle By Name(w972) -> ("median"=w981:dbl, "Phase"=w966:dbl)
            "72 Co Beac" <- w966
            n439 = Negate(x=w1007) -> (-x=w960:dbl)
            "Peak Location Cal" <- w960
            n440 = call "CombineSpectrumAndMedian.vi"("SNR_Thresh"=w978, "median"=w981, "PwrSpectrum"=w980) -> ("Array"=→"Beacon":dbl[][])  [unwired: 8 in]
            n441 = call "PhaseCalculationCount.vi"("Phase"=w966) -> ("PhaseCount"=→"PhaseCount 1":u64)  [unwired: 10 in]
            n442 = Build Array(w983) -> (w984:dbl[])
            n443 = Bundle(w960, w970, w971) -> (→"Freq History 72 Co":cluster{dbl, dbl, dbl})  [unwired: 1 in]
            n444 = local read "NoiseFloorSum"() -> (w1000:dbl)
            n445 = call "PersistentMaxAndMin.vi"("Reset?"="Reset?", "TimeDomainI"=w984) -> ("Numeric"=→"Min":dbl, "Numeric 2"=→"Max":dbl)  [unwired: 8 in]
            n446 = Divide(x=w960, y=1000000.0 ("x")) -> (x/y=→"72CoCalFrq":dbl)
            n447 = Divide(x=w970, y=1000000.0 ("x")) -> (x/y=→"72CoBeacFrq":dbl)
            n448 = Unbundle By Name(w972) -> ("ISpect"=w975:dbl[], "QSpect"=w974:dbl[])
            n449 = call "BuildHistoryCluster.vi"("NewValueWeighting"="NewValueWeighting", "NoiseFloorSum"=w1000, "Channel Power Beac"=w995, "Channel Power Cal"=w968) -> ("output cluster"=w959:T13)  [unwired: 7 in]
            "Power History 72 Co" <- w959
            n450 = Bundle("ISpect"=w975, "QSpect"=w974) -> (→"XY Graph 2":cluster{"ISpect":dbl[], "QSpect":dbl[]})  [unwired: 1 in]
            n451 = control-ref of="Shift Beac"() -> (w998:refnum<vi>)
            n452 = control-ref of="Shift Cal"() -> (w999:refnum<vi>)
            n453 = Bundle By Name(cluster=w1001, "Spectrum 1"=w980, "HistoryWeighting"="NewValueWeighting", "PwrHist.72Co"=w959) -> (w1002:T24)
            n454 = call "OverWriteManualShiftValues.vi"("AutoCenter"=w997, "Shift Beac Val"=w971, "Shift Beac Ref"=w998, "Shift Cal Val"=w969, "Shift Cal Ref"=w999) -> ()  [unwired: 7 in]
          }
          frame "2", Default {
            n455 = Unbundle By Name(w1042) -> ("Cal"=w1041:T57, "Beac"=w1040:T57)
            n456 = Unbundle By Name(w1040) -> ("Shift_"=w1039:dbl, "MaxValue"=w1031:dbl, "Tone"=w1026:T58, "TimeDomainI"=→"TimeDomainBeacon 2":ext[], "PwrSpectrum"=w1032:dbl[], "SNR"=→"SNR 2":dbl, "Tone.DeltaPhase"=→"Delta Phase 72 GHz":dbl, "I_Index"=→"X I_Index":ext[])
            "Beacon 2" <- w1032
            "Channel Power Beac 2" <- w1031
            n457 = Unbundle By Name(w1041) -> ("Shift_"=w1038:dbl, "MaxValue"=w1018:dbl, "Tone"=w1027:T58, "TimeDomainI"=→"TimeDomainCal 2":ext[], "PwrSpectrum"=→"Cal 2":dbl[])
            "Channel Power Cal 2" <- w1018
            "MaxValue_Cal_72X" <- w1018
            n458 = Unbundle By Name(w1027) -> ("PkLocTrak"=w1036:dbl)  [unwired: 1 out]
            n459 = Negate(x=w1038) -> (-x=→"CalShift 2":dbl)
            n460 = Unbundle By Name(w1026) -> ("PkLocDisp"=w1037:dbl)
            n461 = Negate(x=w1039) -> (-x=w1022:dbl)
            "BeaconShift 2" <- w1022
            n462 = Unbundle By Name(w1026) -> ("Phase"=w1016:dbl)
            "72 X Beac" <- w1016
            n463 = Negate(x=w1036) -> (-x=w1019:dbl)
            "Peak Location Cal 2" <- w1019
            n464 = Negate(x=w1037) -> (-x=w1020:dbl)
            "Peak Location Beacon 2" <- w1020
            n465 = call "PhaseCalculationCount.vi"("Phase"=w1016) -> ("PhaseCount"=→"PhaseCount 2":u64)  [unwired: 10 in]
            n466 = Unbundle By Name(w1029) -> ("HistoryWeighting"=w1028:dbl)
            n467 = Bundle(w1019, w1020, w1022) -> (→"Freq History 72 X":cluster{dbl, dbl, dbl})  [unwired: 1 in]
            n468 = local read "NoiseFloorSum 2"() -> (w1030:dbl)
            n469 = call "BuildHistoryCluster.vi"("NewValueWeighting"=w1028, "NoiseFloorSum"=w1030, "Channel Power Beac"=w1031, "Channel Power Cal"=w1018) -> ("output cluster"=w1014:T13)  [unwired: 7 in]
            "Power History 72 X" <- w1014
            n470 = Bundle By Name(cluster=w1029, "Spectrum 2"=w1032, "PwrHist.72X"=w1014) -> (w1033:T24)
          }
          frame "3" {
            # "Disdrometer device resets every 90 days UNLESS signal is too low. Using a variable\nbecause there is no other mechanism for sending data to Disdrometer"
            n471 = Unbundle By Name(w1091) -> ("Cal"=w1090:T57, "Saturat"=→"84 GHz":T3, "Beac"=w1055:T57)
            n472 = Unbundle By Name(w1055) -> ("Shift_"=w1089:dbl, "MaxValue"=w1078:dbl, "Tone"=w1061:T58, "TimeDomainI"=→"TimeDomain Beac 3":ext[], "PwrSpectrum"=w1068:dbl[], "ISpectPos"=→"I Pos":dbl[], "ISpectNeg"=→"I Neg":dbl[], "QSpectPos"=→"Q Pos":dbl[], "QSpectNeg"=→"Q Neg":dbl[], "Tone.ZoomPwr"=→"Power 2":dbl[], "SNR"=w1057:dbl)
            "Channel Power Beac 3" <- w1078
            "SNR 3" <- w1057
            n473 = Unbundle By Name(w1090) -> ("ISpectPos"=→"InPhase Spect":dbl[], "QSpectPos"=→"QuadratureSpect":dbl[], "Shift_"=w1088:dbl, "MaxValue"=w1056:dbl, "Tone"=w1069:T58, "TimeDomainI"=→"TimeDomainCal 3":ext[], "PwrSpectrum"=→"Cal 3":dbl[])  [unwired: 1 out]
            "Channel Power Cal 3" <- w1056
            "MaxValue_Cal_84Co" <- w1056
            n474 = Unbundle By Name(w1061) -> ("PkLocDisp"=w1087:dbl)
            n475 = Unbundle By Name(w1061) -> ("Phase"=w1050:dbl, "median"=w1066:dbl)
            "84 Co Beac" <- w1050
            n476 = Unbundle By Name(w1069) -> ("PkLocTrak"=w1086:dbl)  [unwired: 1 out]
            n477 = Negate(x=w1089) -> (-x=w1058:dbl)
            "BeaconShift 3" <- w1058
            n478 = Negate(x=w1088) -> (-x=w1082:dbl)
            "CalShift 3" <- w1082
            n479 = Negate(x=w1087) -> (-x=w1048:dbl)
            "Peak Location Beacon 3" <- w1048
            n480 = Negate(x=w1086) -> (-x=w1046:dbl)
            "Peak Location Cal 3" <- w1046
            n481 = call "PhaseCalculationCount.vi"("Phase"=w1050) -> ("PhaseCount"=→"PhaseCount 3":u64)  [unwired: 10 in]
            n482 = shared-variable ".\\Disdrometer_Vars.lvlib\\Disdrom_SNR"(w1057) -> ()  [unwired: 1 in, 1 out]
            n483 = Divide(x=w1046, y=1000000.0 ("x")) -> (x/y=→"84CoCalFrq":dbl)
            n484 = call "CombineSpectrumAndMedian.vi"("SNR_Thresh"=w1067, "median"=w1066, "PwrSpectrum"=w1068) -> ("Array"=→"Beacon 3":dbl[][])  [unwired: 8 in]
            n485 = Divide(x=w1048, y=1000000.0 ("x")) -> (x/y=→"84CoBeacFrq":dbl)
            n486 = Bundle(w1046, w1048, w1058) -> (→"Freq History 84 Co":cluster{dbl, dbl, dbl})  [unwired: 1 in]
            n487 = local read "NoiseFloorSum 2"() -> (w1077:dbl)
            n488 = Unbundle By Name(w1076) -> ("HistoryWeighting"=w1075:dbl)
            n489 = Unbundle By Name(w1061) -> ("ISpect"=w1064:dbl[], "QSpect"=w1063:dbl[])
            n490 = call "BuildHistoryCluster.vi"("NewValueWeighting"=w1075, "NoiseFloorSum"=w1077, "Channel Power Beac"=w1078, "Channel Power Cal"=w1056) -> ("output cluster"=w1043:T13)  [unwired: 7 in]
            "Power History 84 Co" <- w1043
            n491 = Bundle("ISpect"=w1064, "QSpect"=w1063) -> (→"XY Graph":cluster{"ISpect":dbl[], "QSpect":dbl[]})  [unwired: 1 in]
            n492 = control-ref of="Shift Cal 3"() -> (w1081:refnum<vi>)
            n493 = control-ref of="Shift Beac 3"() -> (w1080:refnum<vi>)
            n494 = Bundle By Name(cluster=w1076, "Spectrum 3"=w1068, "PwrHist.84Co"=w1043) -> (w1084:T24)
            n495 = call "OverWriteManualShiftValues.vi"("AutoCenter"=w1079, "Shift Beac Val"=w1058, "Shift Beac Ref"=w1080, "Shift Cal Val"=w1082, "Shift Cal Ref"=w1081) -> ()  [unwired: 7 in]
          }
          frame "4" {
            n496 = Unbundle By Name(w1122) -> ("Cal"=w1121:T57, "Beac"=w1120:T57)
            n497 = Unbundle By Name(w1120) -> ("Shift_"=w1119:dbl, "MaxValue"=w1110:dbl, "Tone"=w1105:T58, "TimeDomainI"=→"TimeDomainBeacon 4":ext[], "PwrSpectrum"=w1113:dbl[], "SNR"=→"SNR 4":dbl, "Tone.DeltaPhase"=→"Delta Phase 84 GHz":dbl)
            "Beacon 4" <- w1113
            "Channel Power Beac 4" <- w1110
            n498 = Unbundle By Name(w1121) -> ("Shift_"=w1118:dbl, "MaxValue"=w1098:dbl, "Tone"=w1106:T58, "TimeDomainI"=→"TimeDomainCal 4":ext[], "PwrSpectrum"=→"Cal 4":dbl[])
            "Channel Power Cal 4" <- w1098
            "MaxValue_Cal_84X" <- w1098
            n499 = Unbundle By Name(w1105) -> ("Phase"=w1096:dbl)
            "84 X Beac" <- w1096
            n500 = Negate(x=w1119) -> (-x=w1101:dbl)
            "BeaconShift 4" <- w1101
            n501 = Unbundle By Name(w1105) -> ("PkLocDisp"=w1117:dbl)
            n502 = Unbundle By Name(w1106) -> ("PkLocTrak"=w1116:dbl)
            n503 = Negate(x=w1118) -> (-x=→"CalShift 4":dbl)
            n504 = call "PhaseCalculationCount.vi"("Phase"=w1096) -> ("PhaseCount"=→"PhaseCount 4":u64)  [unwired: 10 in]
            n505 = Negate(x=w1117) -> (-x=w1099:dbl)
            "Peak Location Beacon 4" <- w1099
            n506 = Negate(x=w1116) -> (-x=w1100:dbl)
            "Peak Location Cal 4" <- w1100
            n507 = Bundle(w1100, w1099, w1101) -> (→"Freq History 84 X":cluster{dbl, dbl, dbl})  [unwired: 1 in]
            n508 = Unbundle By Name(w1108) -> ("HistoryWeighting"=w1107:dbl)
            n509 = local read "NoiseFloorSum 2"() -> (w1109:dbl)
            n510 = call "BuildHistoryCluster.vi"("NewValueWeighting"=w1107, "NoiseFloorSum"=w1109, "Channel Power Beac"=w1110, "Channel Power Cal"=w1098) -> ("output cluster"=w1093:T13)  [unwired: 7 in]
            "Power History 84 X" <- w1093
            n511 = Bundle By Name(cluster=w1108, "Spectrum 4"=w1113, "PwrHist.84X"=w1093) -> (w1115:T24)
            n512 = for {
              tunnel: w1094 -> [w1125]
              tunnel: cluster{"Enum":T28, "Data":variant}[] [{"Enum"=enum."FP_Scale", "Data"=variant}, {"Enum"=enum."FP_PWR_Hist", "Data"=variant}] ("element") -> [w1124] mode=indexing
              n513 = Enqueue Element(queue=w1125, element=w1124, timeout in ms (-1)=10) -> ()  [unwired: 1 in, 3 out]
            }
          }
        }
      }
      frame "FP_Noise" {
        # "From Noise_Send"
        n514 = Variant To Data(error in=w1133, type=cluster{"Target":T21, "1":T59} {"Target"=enum."1", "1"={"df"=0.0, "AvgAvgSpectrum"=[], "FFT_Index"=[], "Avg'd"=[], "Sum"=0.0, "SumdSpectrum"=[], "SumCount"=0}} ("cluster"), Variant=w1132) -> (data=w1131:cluster{"Target":T21, "1":T59})  [unwired: 1 out]
        n515 = Unbundle(w1131) -> ("Target"=w1130:T21, "1"=w1129:T59)
        n516 = case shown="\"4\"" w1130 {
          tunnel: w1129 -> [w1140 w1145 w1150 w1155]
          tunnel: w1127 -> [w1137 w1143 w1148 w1153]
          tunnel: [w1135 w1142 w1147 w1152] -> w1126
          frame "1", Default {
            n517 = Unbundle By Name(w1140) -> ("df"=→"df (Hz)":dbl, "AvgAvgSpectrum"=→"NoiseFloor":dbl[], "Sum"=w1136:dbl)  [unwired: 2 out]
            "NoiseFloorSum" <- w1136
            n518 = Bundle By Name(cluster=w1137, "NoiseFloorSums.1"=w1136) -> (w1135:T24)
            n519 = Unbundle By Name(w1135) -> ("NoiseFloorSums"=→"Noise Floor Sum Histories":T25)
          }
          frame "2" {
            n520 = Unbundle By Name(w1145) -> ("AvgAvgSpectrum"=→"NoiseFloor 2":dbl[], "Sum"=w1141:dbl)  [unwired: 3 out]
            "NoiseFloorSum 2" <- w1141
            n521 = Bundle By Name(cluster=w1143, "NoiseFloorSums.2"=w1141) -> (w1142:T24)
          }
          frame "3" {
            n522 = Unbundle By Name(w1150) -> ("AvgAvgSpectrum"=→"NoiseFloor 3":dbl[], "Sum"=w1146:dbl)  [unwired: 3 out]
            "NoiseFloorSum 3" <- w1146
